vi "RampPressure_v01.vi"(2 "Debug Mode":bool, 3 "Elapsed Time(s)":dbl, 4 "State":enum16{"Edit", "Start", "Run", "End", "Idle"}(ring), 5 "Argument List In":string[](array[string])) -> (0 "Status Out":string, 1 "Argument List Out":string[](array[string]))   [LabVIEW 2011]
panel:
  out "error out":errorcluster
  in  "P initial (torr)":dbl
  in  "P current":dbl
  in  "ramp time (s)":dbl=20.0 format="%.1f"
  in  "Set Point":string(combo)="C"
  in  "P final (torr)":dbl=20.0 format="%.1f"
  out "total time":dbl
  out "is OK?":bool
  in  "Cancel":bool
  in  "OK":bool
  out "tTotal(s) 2":dbl
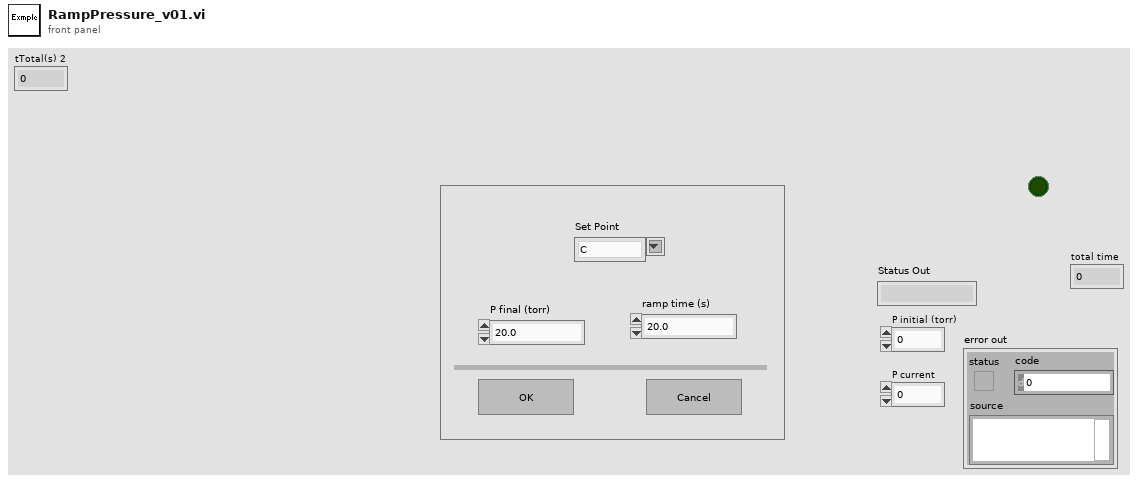
[diagram p1: front panel]
types:
  T1 = enum16{"Discrete", "Continuous", "Instantaneous", "Finite"}
  T2 = enum32{"Invalid", "Default", "Floating", "Floating/Auto-Hide", "Modal"}
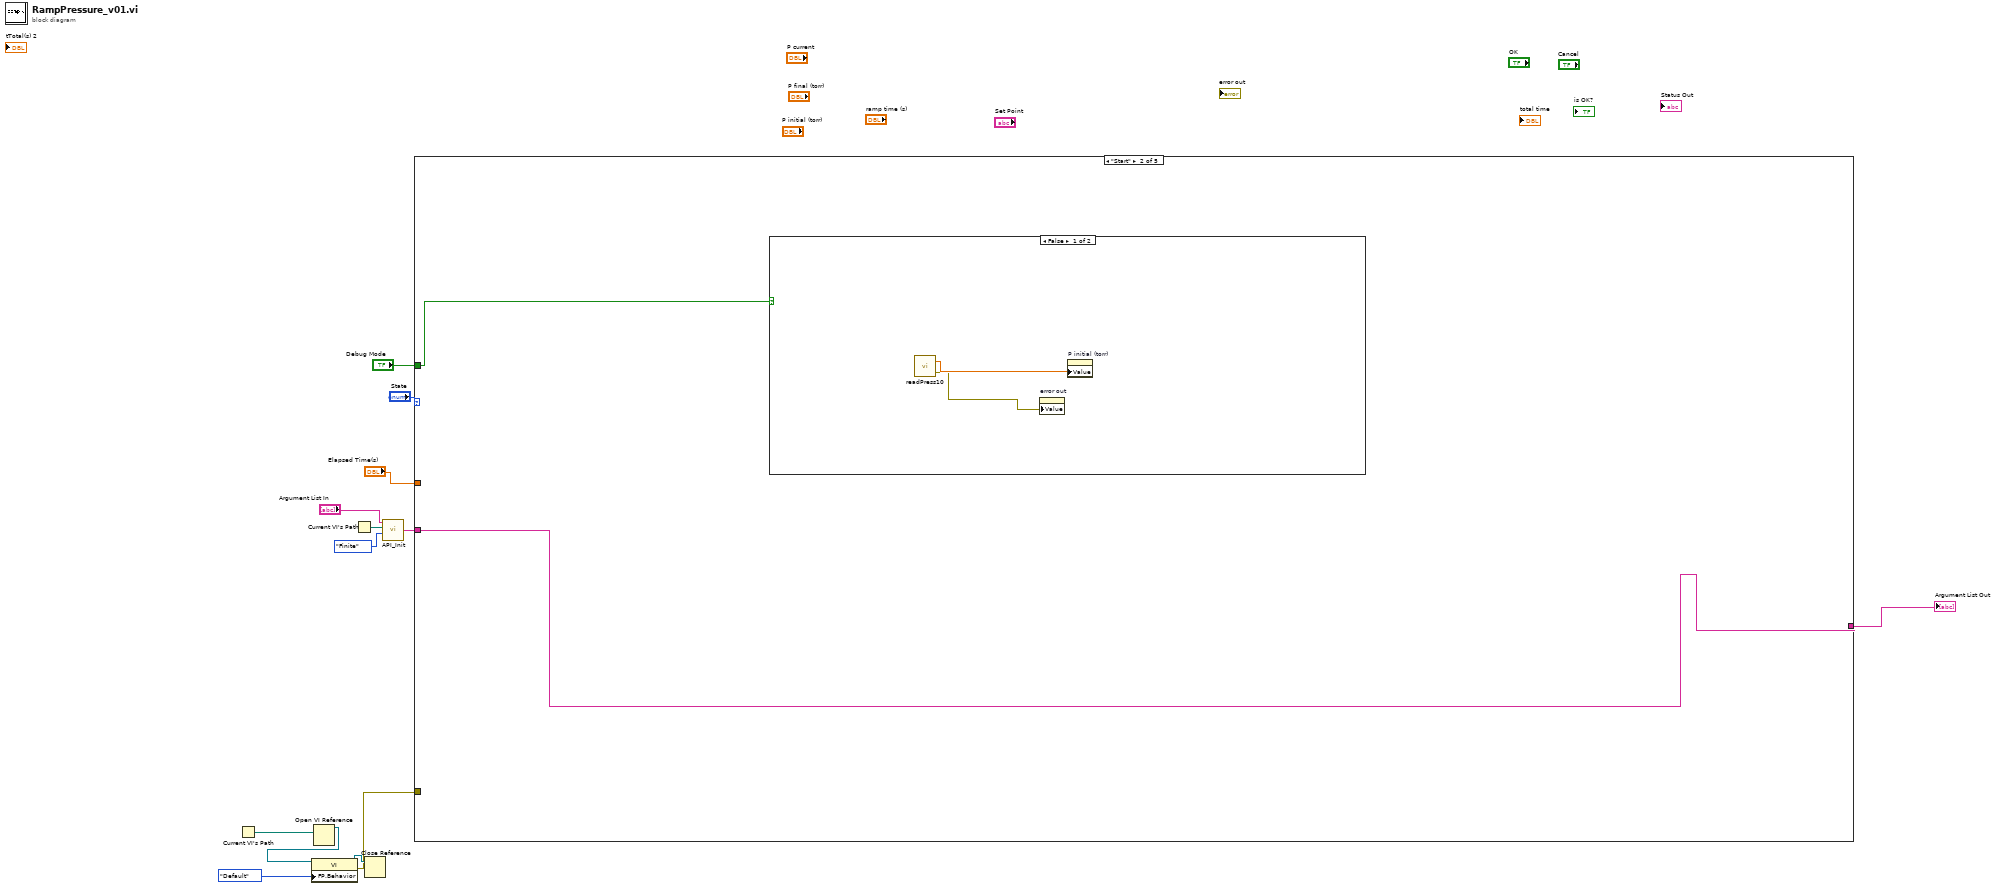
[diagram p0: block diagram]
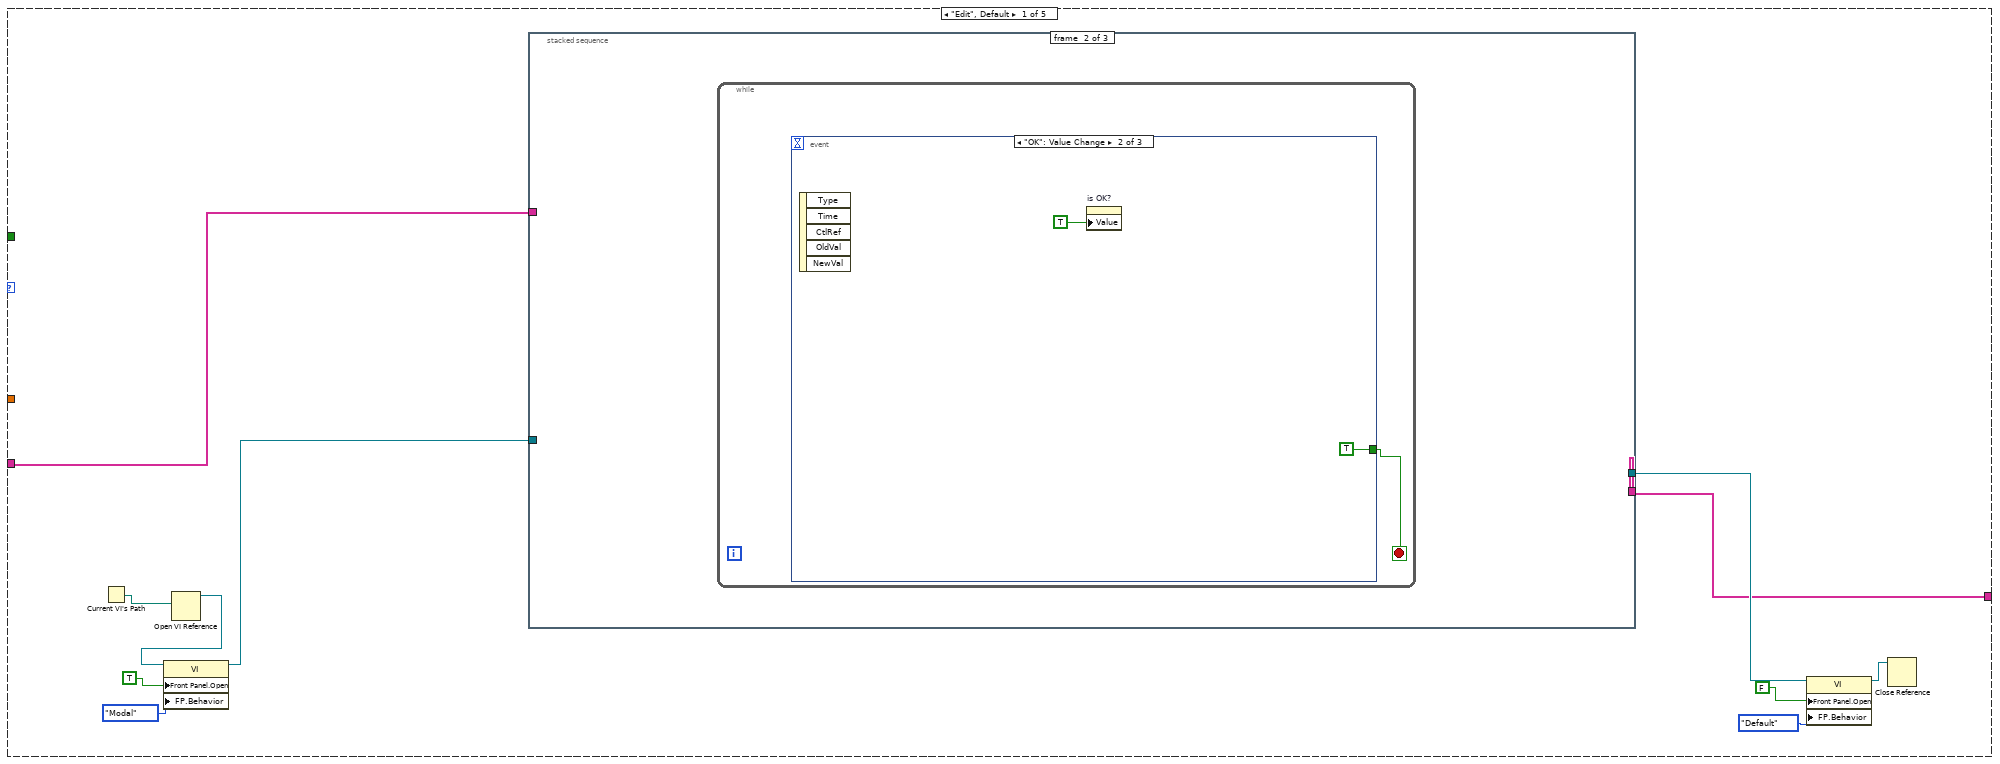
[diagram p2: hidden frame]
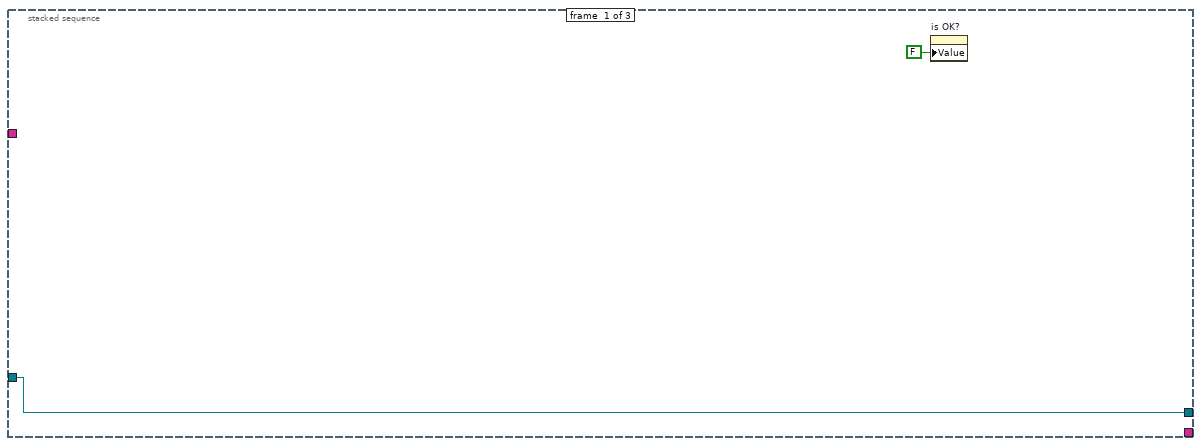
[diagram p3: hidden frame]
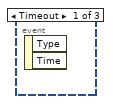
[diagram p4: hidden frame]
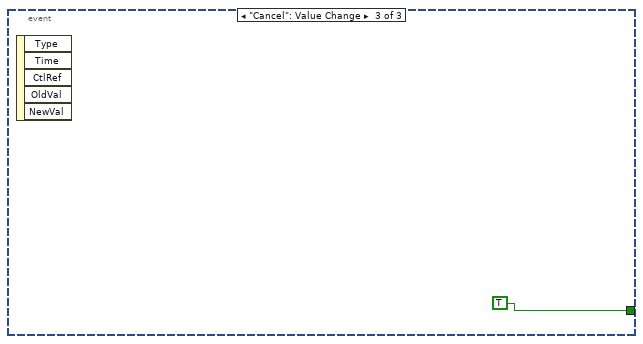
[diagram p5: hidden frame]
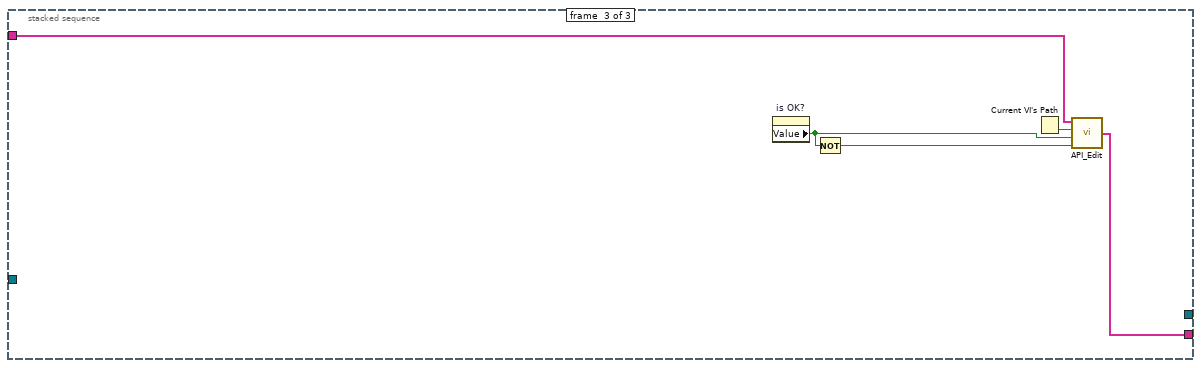
[diagram p6: hidden frame]
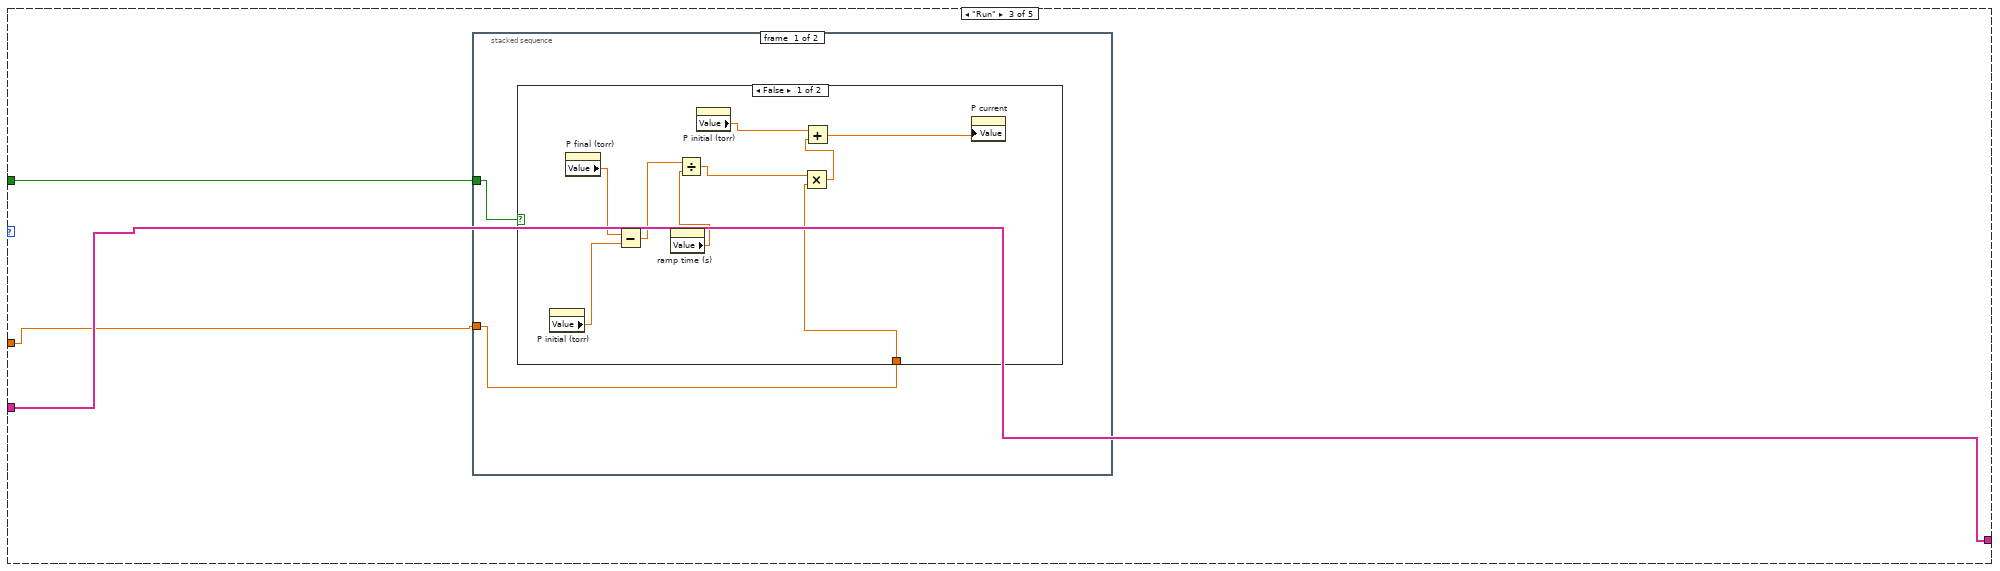
[diagram p8: hidden frame]
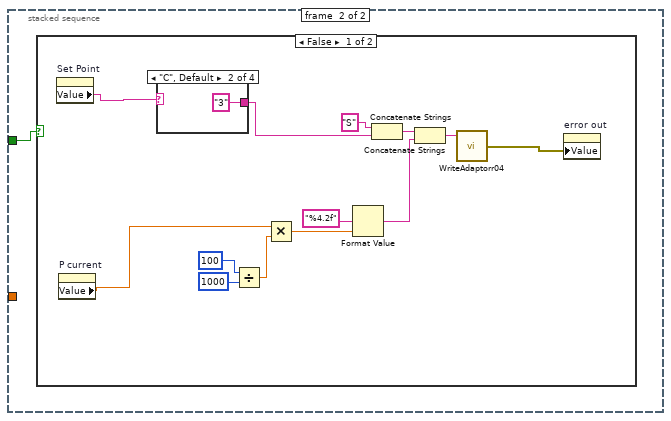
[diagram p10: hidden frame]
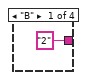
[diagram p11: hidden frame]
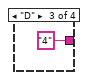
[diagram p12: hidden frame]
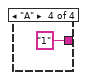
[diagram p13: hidden frame]
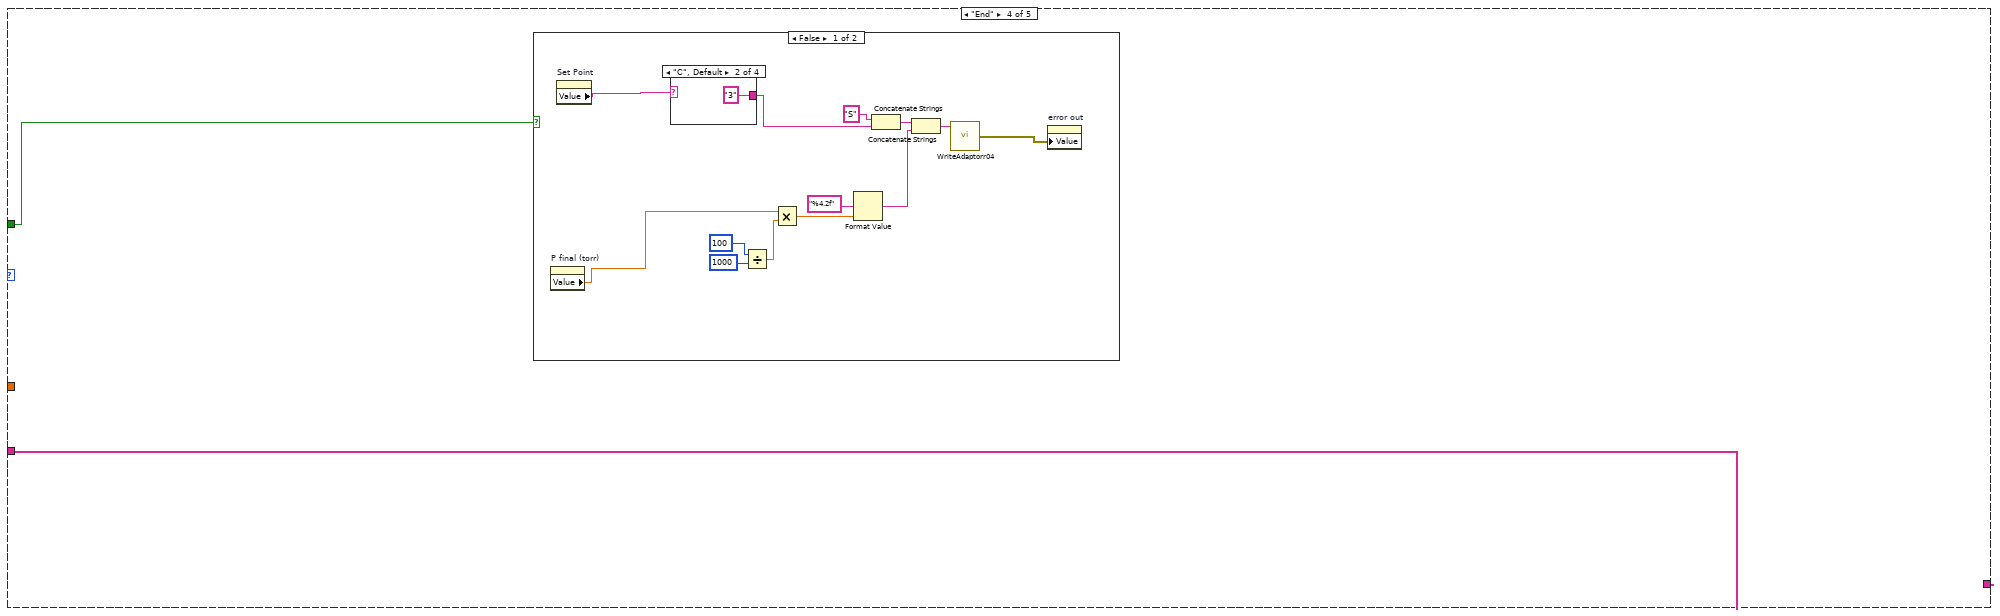
[diagram p15: hidden frame]
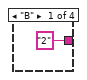
[diagram p16: hidden frame]
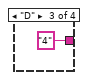
[diagram p17: hidden frame]
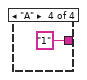
[diagram p18: hidden frame]
diagram:
  n1 = Current VI's Path() -> (path=w9:path)
  n2 = Open VI Reference(vi path=w9) -> (vi reference=w8:refnum<vi>)  [unwired: 1 in, 5 out]
  n3 = property class="VI"(reference=w8, "FP.Behavior"=T2."Default" ("Front Panel Window:Behavior")) -> (reference out=w6:refnum<vi>, error out=w5:errorcluster)  [unwired: 1 in]
  n4 = Current VI's Path() -> (path=w4:path)
  n5 = Close Reference(reference=w6) -> ()  [unwired: 1 in, 1 out]
  n6 = call "API_Init.vi"("API Mode"=T1."Finite", "VI Path"=w4, "Argument List In"="Argument List In") -> ("Argument List Out"=w1:string[])  [unwired: 1 in]
  n7 = case shown="\"Start\"" "State" {
    tunnel: "Debug Mode" -> [_ w36 w40 w72 _]
    tunnel: "Elapsed Time(s)" -> [_ _ w41 _ _]
    tunnel: w1 -> [w15 w37 w42 w73 w91]
    tunnel: [w14 w37 w42 w73 w91] -> w10
    tunnel: w5 -> [_ _ _ _ _]
    frame "Edit", Default {
      n8 = Current VI's Path() -> (path=w20:path)
      n9 = Open VI Reference(vi path=w20) -> (vi reference=w19:refnum<vi>)  [unwired: 1 in, 5 out]
      n10 = property class="VI"(reference=w19, "Front Panel.Open"=TRUE ("Front Panel Window:Open"), "FP.Behavior"=T2."Modal" ("Front Panel Window:Behavior")) -> (reference out=w18:refnum<vi>)  [unwired: 1 in, 1 out]
      n11 = stacked-sequence {
        tunnel: w15 -> [_ _ w31]
        tunnel: w18 -> [w26 _ _]
        tunnel: [w26 _ _] -> w22
        tunnel: [_ _ w33] -> w14
        frame #0 {
          n12 = property on="is OK?" class="Bool (strict)"("Value"=FALSE ("is OK?")) -> ()  [unwired: 2 in, 2 out]
        }
        frame #1 {
          n13 = while {
            stop <- w27 stop-if-true
            n14 = event shown="[1] \"OK\": Value Change" {
              selector: _ -> [_ _ _]
              dyn-events: _ -> [_ _ _]
              timeout: _ -> [_ _ _]
              tunnel: [_ TRUE TRUE] -> w27
              event Timeout {
                n15 = event-data() -> ()  [unwired: 1 in, 2 out]
              }
              event "OK": Value Change {
                n16 = event-data() -> ()  [unwired: 1 in, 5 out]
                n17 = property on="is OK?" class="Bool (strict)"("Value"=TRUE ("is OK?")) -> ()  [unwired: 2 in, 2 out]
              }
              event "Cancel": Value Change {
                n18 = event-data() -> ()  [unwired: 1 in, 5 out]
              }
            }
          }
        }
        frame #2 {
          n19 = property on="is OK?" class="Bool (strict)"() -> ("Value"=w32:bool)  [unwired: 2 in, 2 out]
          n20 = Not(x=w32) -> (.not. x?=w35:bool)
          n21 = Current VI's Path() -> (path=w34:path)
          n22 = call "API_Edit.vi"("Cancel"=w35, "OK"=w32, "VI Path"=w34, "Argument List In"=w31) -> ("Argument List Out"=w33:string[])
        }
      }
      n23 = property class="VI"(reference=w22, "Front Panel.Open"=FALSE ("Front Panel Window:Open"), "FP.Behavior"=T2."Default" ("Front Panel Window:Behavior")) -> (reference out=w23:refnum<vi>)  [unwired: 1 in, 1 out]
      n24 = Close Reference(reference=w23) -> ()  [unwired: 1 in, 1 out]
    }
    frame "Start" {
      n25 = case shown="False" w36 {
        frame False {
          n26 = call "readPress10.vi"() -> ("P"=w39:dbl, "error out"=w38:errorcluster)  [unwired: 1 in]
          n27 = property on="error out" class="Clust (strict)"("Value"=w38) -> ()  [unwired: 2 in, 2 out]
          n28 = property on="P initial (torr)" class="DigNum (strict)"("Value"=w39) -> ()  [unwired: 2 in, 2 out]
        }
        frame True {
        }
      }
    }
    frame "Run" {
      n29 = stacked-sequence {
        tunnel: w41 -> [w44 _]
        tunnel: w40 -> [w43 w54]
        frame #0 {
          n30 = case shown="False" w43 {
            tunnel: w44 -> [w47 _]
            frame False {
              n31 = property on="P initial (torr)" class="DigNum (strict)"() -> ("Value"=w52:dbl)  [unwired: 2 in, 2 out]
              n32 = property on="P final (torr)" class="DigNum (strict)"() -> ("Value"=w53:dbl)  [unwired: 2 in, 2 out]
              n33 = Subtract(x=w53, y=w52) -> (x-y=w51:dbl)
              n34 = property on="ramp time (s)" class="DigNum (strict)"() -> ("Value"=w50:dbl)  [unwired: 2 in, 2 out]
              n35 = Divide(x=w51, y=w50) -> (x/y=w46:dbl)
              n36 = property on="P initial (torr)" class="DigNum (strict)"() -> ("Value"=w49:dbl)  [unwired: 2 in, 2 out]
              n37 = Multiply(x=w46, y=w47) -> (x*y=w48:dbl)
              n38 = Add(x=w49, y=w48) -> (x+y=w45:dbl)
              n39 = property on="P current" class="DigNum (strict)"("Value"=w45) -> ()  [unwired: 2 in, 2 out]
            }
            frame True {
            }
          }
        }
        frame #1 {
          n40 = case shown="False" w54 {
            frame False {
              n41 = property on="Set Point" class="CmbBox"() -> ("Value"=w57:string)  [unwired: 2 in, 2 out]
              n42 = property on="P current" class="DigNum (strict)"() -> ("Value"=w56:dbl)  [unwired: 2 in, 2 out]
              n43 = case shown="\"C\", Default" w57 {
                tunnel: ["2" "3" "4" "1"] -> w58
                frame "B" {
                }
                frame "C", Default {
                }
                frame "D" {
                }
                frame "A" {
                }
              }
              n44 = Divide(x=100, y=1000) -> (x/y=w63:dbl)
              n45 = Multiply(x=w56, y=w63) -> (x*y=w66:dbl)
              n46 = Format Value(format string="%4.2f", value (0)=w66) -> (output string=w67:string)  [unwired: 1 in]
              n47 = Concatenate Strings("S", w58) -> (w59:string)
              n48 = Concatenate Strings(w59, w67) -> (w64:string)
              n49 = call "WriteAdaptorr04.vi"("string to write"=w64) -> ("error out"=w55:errorcluster)  [unwired: 2 in]
              n50 = property on="error out" class="Clust (strict)"("Value"=w55) -> ()  [unwired: 2 in, 2 out]
            }
            frame True {
            }
          }
        }
      }
    }
    frame "End" {
      n51 = case shown="False" w72 {
        frame False {
          n52 = property on="P final (torr)" class="DigNum (strict)"() -> ("Value"=w74:dbl)  [unwired: 2 in, 2 out]
          n53 = property on="Set Point" class="CmbBox"() -> ("Value"=w76:string)  [unwired: 2 in, 2 out]
          n54 = case shown="\"C\", Default" w76 {
            tunnel: ["2" "3" "4" "1"] -> w77
            frame "B" {
            }
            frame "C", Default {
            }
            frame "D" {
            }
            frame "A" {
            }
          }
          n55 = Divide(x=100, y=1000) -> (x/y=w82:dbl)
          n56 = Multiply(x=w74, y=w82) -> (x*y=w85:dbl)
          n57 = Format Value(format string="%4.2f", value (0)=w85) -> (output string=w86:string)  [unwired: 1 in]
          n58 = Concatenate Strings("S", w77) -> (w78:string)
          n59 = Concatenate Strings(w78, w86) -> (w83:string)
          n60 = call "WriteAdaptorr04.vi"("string to write"=w83) -> ("error out"=w75:errorcluster)  [unwired: 2 in]
          n61 = property on="error out" class="Clust (strict)"("Value"=w75) -> ()  [unwired: 2 in, 2 out]
        }
        frame True {
        }
      }
    }
    frame "Idle" {
    }
  }
  "Argument List Out" <- w10
